vi "Read Compatibility Helper Type.vi"(11 "Test Executive Builder Model in":refnum<class "Test Executive Builder Model.lvclass">) -> (2 "Compatibility Helper":refnum<class "ICompatibility Helper.lvclass">, 3 "Test Executive Builder Model out":refnum<class "Test Executive Builder Model.lvclass">)   [LabVIEW 2017, in "Test Executive Builder Model.lvclass"]
uses:
  Test Executive Builder Model.lvclass
  <vilib>/gpm_packages/@cs/test-executive/Source/Compatibility Helper/ICompatibility Helper.lvclass
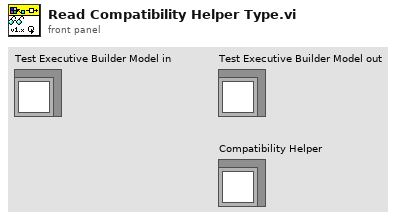
[diagram p1: front panel]
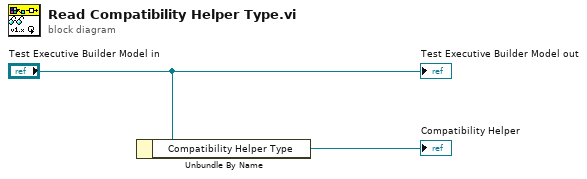
[diagram p0: block diagram]
diagram:
  n1 = Unbundle By Name("Test Executive Builder Model in") -> ("Compatibility Helper Type"=→"Compatibility Helper":refnum<class "ICompatibility Helper.lvclass">)
  "Test Executive Builder Model out" <- "Test Executive Builder Model in"
